vi "integrate.vi"(5 "waiting iterations per pixel":u32, 7 "integration iterations per pixel":u32, 9 "iteration counter in":u32, 10 "sampling values in":T1, 11 "previous pixel values in":T1) -> (1 "finished?":bool, 2 "iteration counter out":u32, 3 "new pixel values out":T1)   [LabVIEW 2011]
uses:
  typedefs/channels_array.ctl
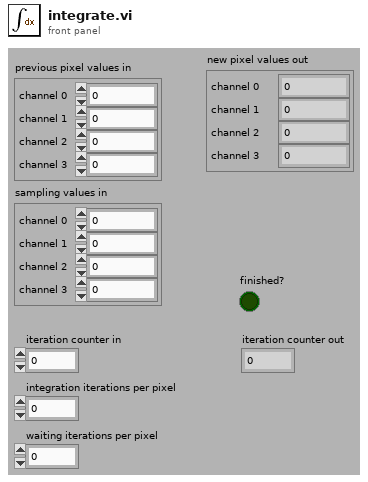
[diagram p1: front panel]
types:
  T1 = typedef "channels_array.ctl" = cluster{"channel 0":u32, "channel 1":u32, "channel 2":u32, "channel 3":u32}
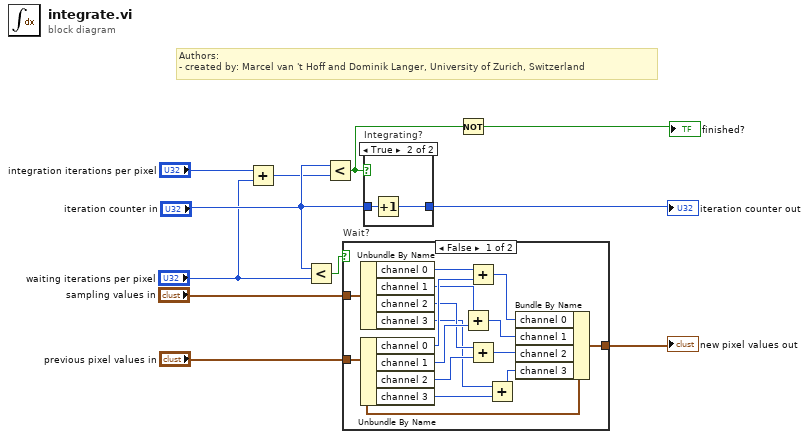
[diagram p0: block diagram]
diagram:
  # "Authors: \n- created by: Marcel van 't Hoff and Dominik Langer, University of Zurich, Switzerland"
  n1 = Add(x="integration iterations per pixel", y="waiting iterations per pixel") -> (x+y=w2:u32)
  n2 = Less?(x="iteration counter in", y="waiting iterations per pixel") -> (x < y?=w3:bool)
  n3 = Less?(x="iteration counter in", y=w2) -> (x < y?=w1:bool)
  n4 = case "Wait?" shown="False" w3 {
    tunnel: "sampling values in" -> [w18 _]
    tunnel: "previous pixel values in" -> [w17 w27]
    tunnel: [w12 w27] -> w9
    frame False {
      n5 = Unbundle By Name(w18) -> ("channel 0"=w26:u32, "channel 1"=w24:u32, "channel 2"=w22:u32, "channel 3"=w20:u32)
      n6 = Unbundle By Name(w17) -> ("channel 0"=w25:u32, "channel 1"=w23:u32, "channel 2"=w21:u32, "channel 3"=w19:u32)
      n7 = Add(x=w24, y=w23) -> (x+y=w15:u32)
      n8 = Add(x=w26, y=w25) -> (x+y=w16:u32)
      n9 = Add(x=w22, y=w21) -> (x+y=w14:u32)
      n10 = Add(x=w20, y=w19) -> (x+y=w13:u32)
      n11 = Bundle By Name(cluster=w17, "channel 0"=w16, "channel 1"=w15, "channel 2"=w14, "channel 3"=w13) -> (w12:T1)
    }
    frame True {
    }
  }
  "new pixel values out" <- w9
  n12 = case "Integrating?" shown="True" w1 {
    tunnel: [_ w29] -> w7
    tunnel: "iteration counter in" -> [_ w28]
    frame False {
      # "Finished!"
    }
    frame True {
      n13 = Increment(x=w28) -> (x+1=w29:u32)
    }
  }
  "iteration counter out" <- w7
  n14 = Not(x=w1) -> (.not. x?=→"finished?":bool)
